vi "Path-White_Tiles.vi"(10 "Adjacent Tiles":T1[](array[typedef])) -> (1 "White Tiles?":bool, 2 "Tiles":T1[](array[typedef]))   [LabVIEW 2020]
doc: "<B>Description:</B> Checks adjacent tiles for white or red tiles. If there are white or red tiles, only those are returned. Otherwise, all the purple tiles are returned instead.\n\n<B>Date:</B> 05/2019\n<B>Author:</B>Luke Jarocki, Choose Movement Consulting, LLC"
uses:
  Controls/Parse-(X,Y).ctl
  Controls/TileColor.ctl
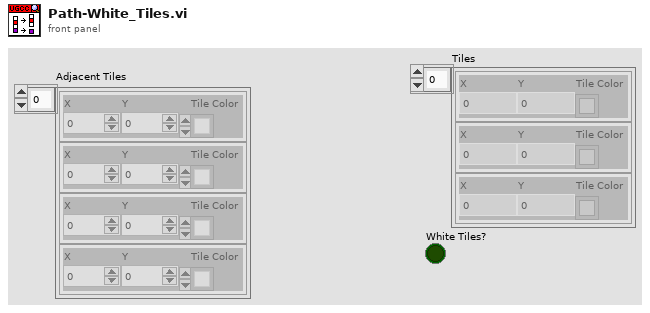
[diagram p1: front panel]
types:
  T1 = typedef "Parse-(X,Y).ctl" = cluster{"X":i32, "Y":i32, "Tile Color":T2}
  T2 = typedef "TileColor.ctl" = u16
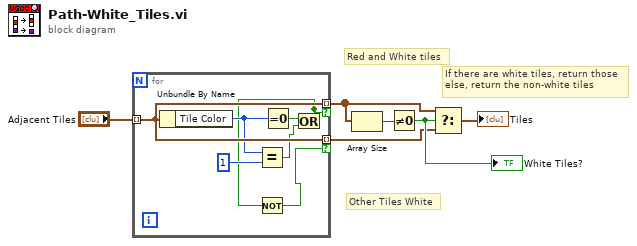
[diagram p0: block diagram]
diagram:
  # "If there are white tiles, return those\nelse, return the non-white tiles"
  # "Other Tiles White"
  # "Red and White tiles"
  n1 = for {
    tunnel: "Adjacent Tiles" -> [w13] mode=indexing
    tunnel: [w13] -> w2 mode=indexing if=w8
    tunnel: [w13] -> w1 mode=indexing if=w7
    n2 = Unbundle By Name(w13) -> ("Tile Color"=w12:T2)
    n3 = Equal?(x=w12, y=T2 1) -> (x = y?=w9:bool)
    n4 = Equal To 0?(x=w12) -> (x = 0?=w10:bool)
    n5 = Or(x=w10, y=w9) -> (x .or. y?=w8:bool)
    n6 = Not(x=w8) -> (.not. x?=w7:bool)
  }
  n7 = Array Size(array=w2) -> (size(s)=w5:i32)
  n8 = Not Equal To 0?(x=w5) -> (x != 0?=w4:bool)
  "White Tiles?" <- w4
  n9 = Select(t=w2, s=w4, f=w1) -> (s? t:f=→"Tiles":T1[])
